vi "Digitizer.vi"() -> ()   [LabVIEW 2021]
uses:
  <vilib>/Platform/TimedLoop/XDataNode/timing_clust.ctl
  <vilib>/Platform/TimedLoop/XDataNode/nitl_modes.ctl
  <vilib>/Platform/TimedLoop/XDataNode/wakeup.ctl
  <vilib>/platform/TimedLoop/XDataNode/XDataNode.xnode
  <vilib>/Platform/TimedLoop/XDataNode/XDNodeRunTimeDep.lvlib
  <userlib>/SciSDK/SciSDK_Labview.lvlib
panel:
  in  "stop":bool
  out "CH1":i32[](graph)
  out "CH0":i32[](graph)
  out "error out":errorcluster
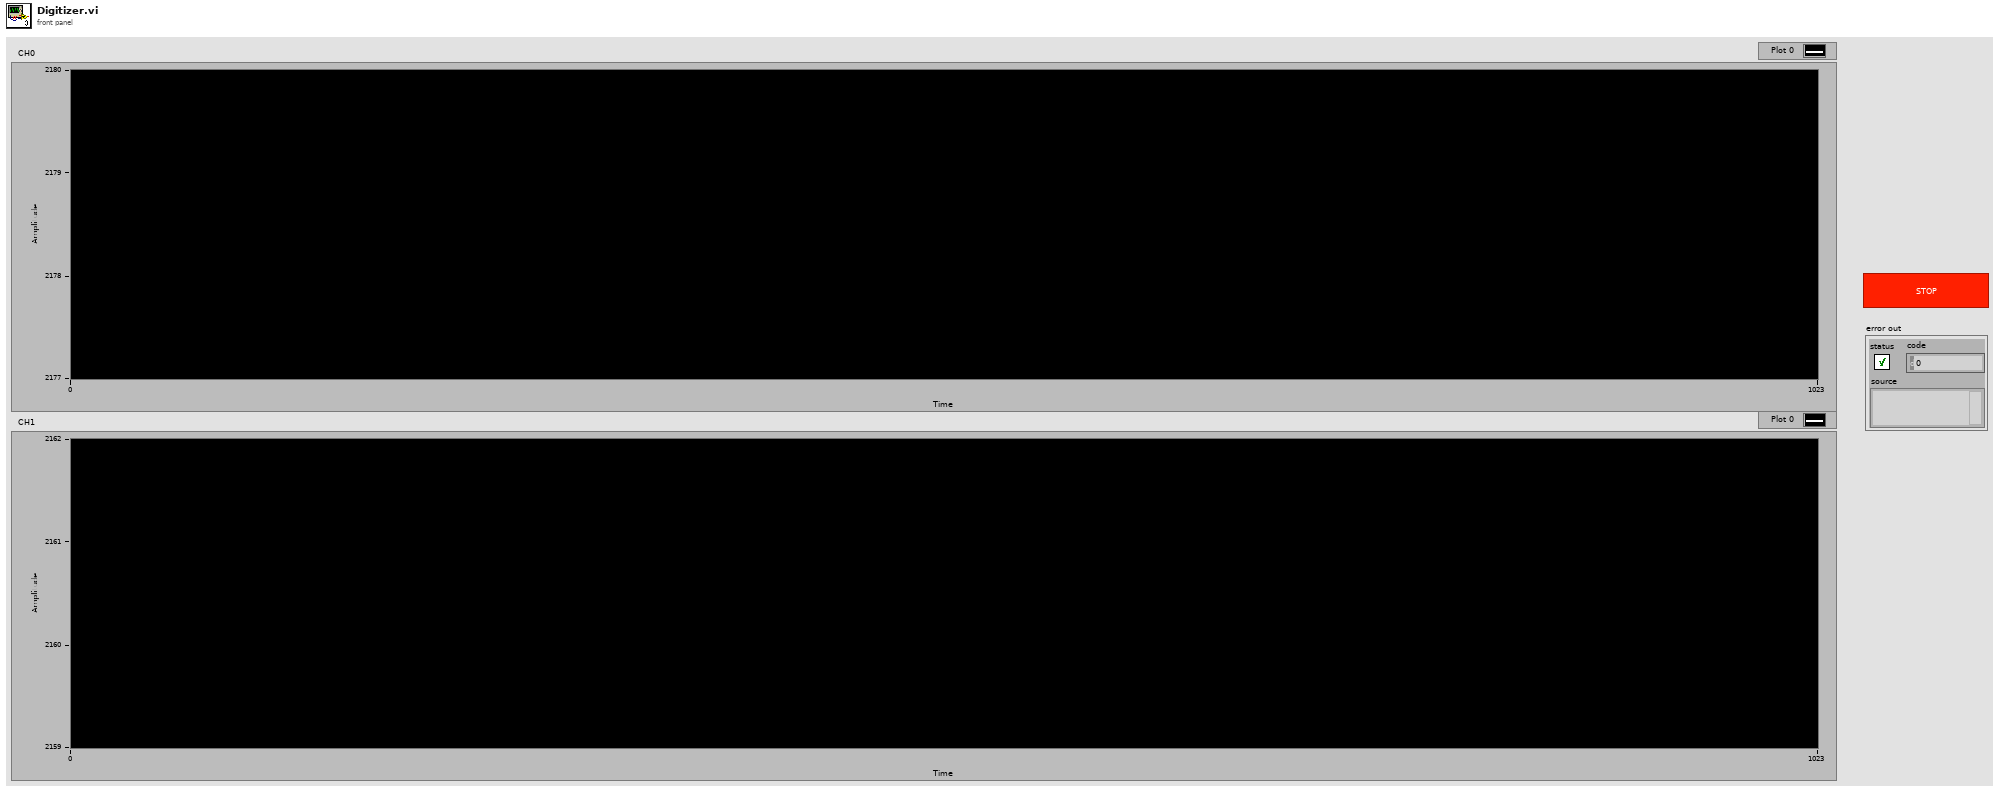
[diagram p1: front panel]
types:
  T1 = cluster{"Name":string, "Board Model":string, "Handle":u64}
  T2 = cluster{"Digitizer Path":string, "Digitizer Name":string}
  T3 = cluster{"Board Name":string, "Board Model":string, "Handle":u64}
  T4 = typedef "XDNodeRunTimeDep.lvlib/timing_clust.ctl" = cluster{"Expected End [f-1]":u64, "Actual End [f-1]":u64, "Finished Late? [f-1]":bool, "Expected End [i-1]":u64, "Actual End [i-1]":u64, "Finished Late? [i-1]":bool, "Expected Start [i]":u64, "Actual Start [i]":u64, "Expected Start [f]":u64, "Actual Start [f]":u64, "Source Name":string, "Structure Name":string, "Period":i64, "Deadline":i64, "Offset":i64, "Start":i64, "Priority":i32, "Timeout":i32, "Mode":T5, "Wakeup Reason":T6, "Error":errorcluster, "Source Type":string, "Secondary Source Type":string, "Global End Time":u64, "Global Start Time":u64, "Frame Duration":u64, "Iteration Duration":u64, "Assigned CPU":i32, "I/O Scan Engine Mode":u32}
  T5 = typedef "XDNodeRunTimeDep.lvlib/nitl_modes.ctl" = enum32{"No Change", "Process missed periods, maintain original phase", "Discard missed periods, maintain original phase", "Process missed periods, ignore original phase", "Discard missed periods, ignore original phase"}
  T6 = typedef "XDNodeRunTimeDep.lvlib/wakeup.ctl" = enum32{"Normal", "Aborted", "Asynchronous wakeup", "Timing source error", "Timed loop error", "Timeout"}
  T7 = cluster{"analog":i32[][], "magic":u32, "hits":u32, "timecode":u32, "counter":u32, "user":u32, "samples":u32, "valid_samples":u32, "channels":u32, "enabled_channels":u32}
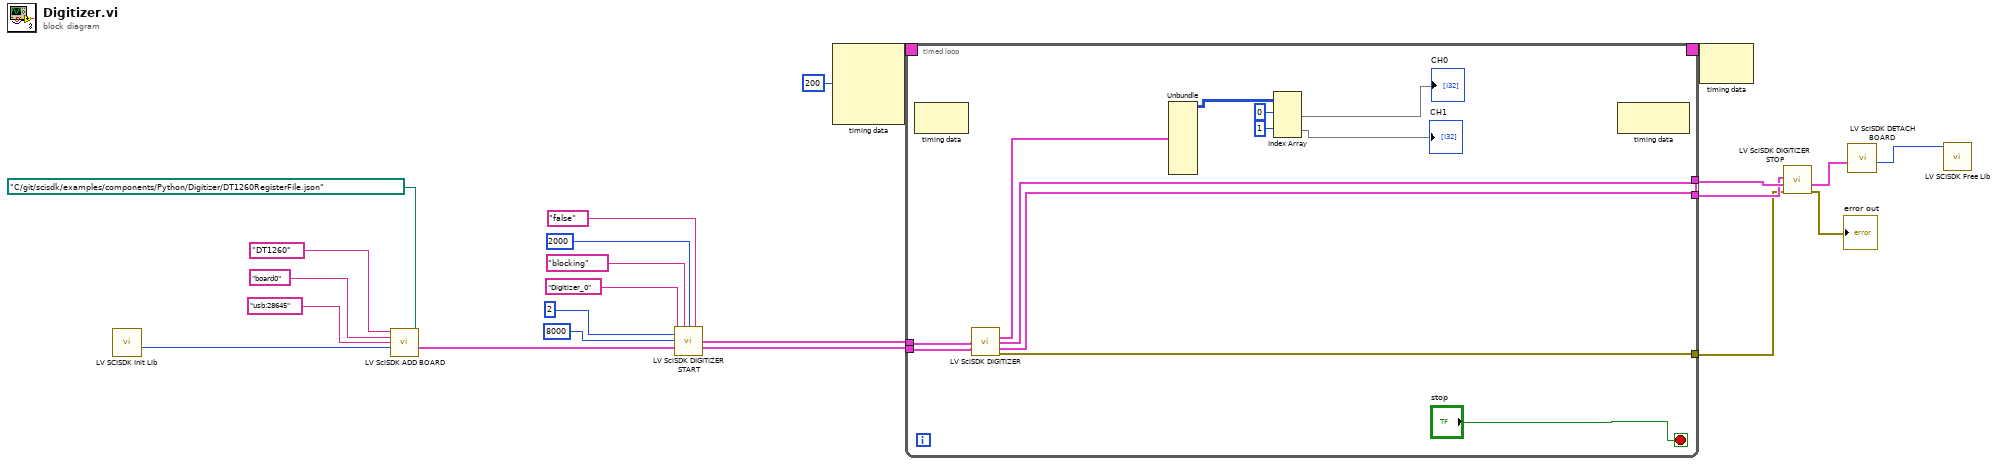
[diagram p0: block diagram]
diagram:
  n1 = call <userlib>:"LV SCISDK Init Lib.vi"() -> ("function return"=w19:u64)  [unwired: 11 in]
  n2 = call <userlib>:"LV SciSDK ADD BOARD.vi"("JsonFile"=path "C:/git/scisdk/examples/components/Python/Digitizer/DT1260RegisterFile.json", "Board Model"="DT1260", "SciSDK Handle"=w19, "DevicePath"="usb:28645", "Name"="board0") -> ("Board Handle Out"=w15:T1)  [unwired: 4 in, 2 out]
  n3 = call <userlib>:"LV SciSDK DIGITIZER START.vi"("Digitizer Name"="Digitizer_0", "Acq mode"="blocking", "Timeout"=2000, "High performance"="false", "Enabled channels"=u32 2, "Acq len"=u32 8000, "Board Handle In"=w15) -> ("Digitizer Handle Out"=w8:T2, "Board Handle Out"=w9:T3)  [unwired: 6 in, 1 out]
  n4 = node-c288(i64 200 ("Period")) -> (w23:T4)  [unwired: 3 in]
  n5 = timed-loop {
    timing: w23 -> [_]
    timing-out: [_] -> w22
    tunnel: w8 -> [w28]
    tunnel: w9 -> [w29]
    tunnel: [w24] -> w6
    tunnel: [w27] -> w4
    tunnel: [w25] -> w5
    stop <- "stop" stop-if-true
    n6 = node-c288() -> ()  [unwired: 1 in, 1 out]
    n7 = call <userlib>:"LV SciSDK DIGITIZER.vi"("Digitizer Handle In"=w28, "Board Handle In"=w29) -> ("Digitizer Buffer Out"=w26:T7, "Digitizer Handle Out"=w25:T2, "Board Handle Out"=w24:T3, "error out"=w27:errorcluster)  [unwired: 9 in, 1 out]
    n8 = Unbundle(w26) -> ("analog"=w35:i32[][])  [unwired: 9 out]
    n9 = Index Array(array=w35, index (row) #1=0 ("index (row)"), index (row) #2=1 ("index (row)")) -> (element #1=→"CH0":i32[], element #2=→"CH1":i32[])  [unwired: 2 in]
    n10 = node-c288() -> ()  [unwired: 1 in, 1 out]
  }
  n11 = node-c288(w22) -> ()  [unwired: 1 out]
  n12 = call <userlib>:"LV SciSDK DIGITIZER STOP.vi"("error in (no error)"=w4, "Board Handle In"=w6, "Digitizer Handle In"=w5) -> ("error out"=→"error out":errorcluster, "Board Handle Out"=w2:T3)  [unwired: 6 in, 1 out]
  n13 = call <userlib>:"LV SciSDK DETACH BOARD.vi"("Board Handle In"=w2) -> ("SciSDK Handle"=w3:u64)  [unwired: 9 in, 1 out]
  n14 = call <userlib>:"LV SCISDK Free Lib.vi"("handle"=w3) -> ()  [unwired: 9 in, 2 out]
